vi "s3_bucket_demo.vi"() -> ()   [LabVIEW 2018]
uses:
  <vilib>/AWS Toolkit/Core/HTTP Request/Region.ctl
  <vilib>/AWS Toolkit/S3/ACL.ctl
  <vilib>/AWS Toolkit/S3/Bucket/Bucket.lvclass
  <vilib>/AWS Toolkit/Core/HTTP Request/AWS Credentials.ctl
  <vilib>/AWS Toolkit/Core/HTTP Request/HTTP Request.lvclass
  <vilib>/AWS Toolkit/S3/NI_AWS_S3.lvlib
panel:
  out "error constant":errorcluster
  out "Enum":T1(ring)
  in  "Stop":bool
  out "Owner display name":string
  out "Owner ID":string
  out "Buckets":refnum<class "Bucket.lvclass">[](array[class])
  in  "Access Control List":T2
  in  "Region":T3
  in  "Bucket Name":string
  in  "List":bool
  in  "Delete":bool
  in  "Create":bool
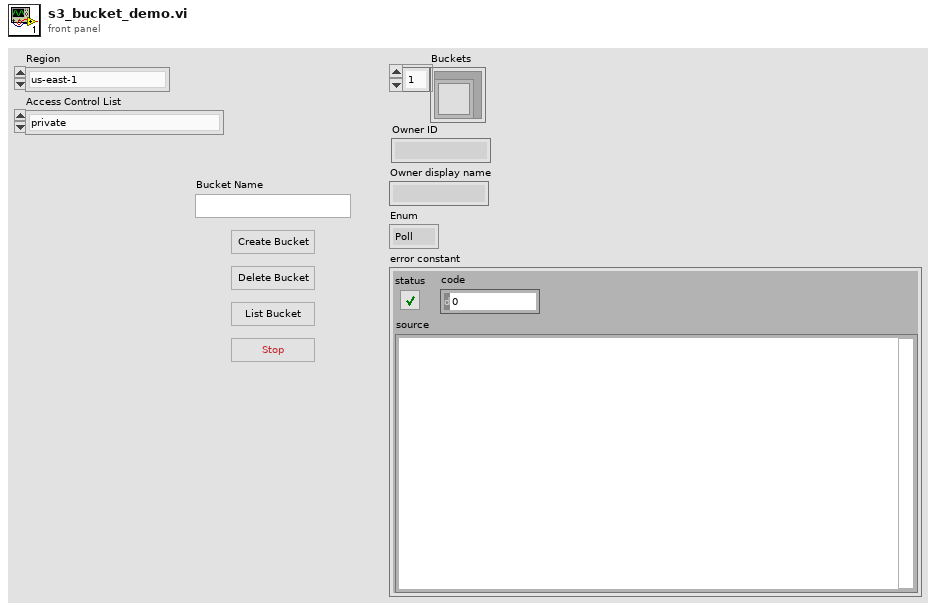
[diagram p1: front panel]
types:
  T1 = enum16{"Poll", "Create", "List", "Delete", "Shutdown"}
  T2 = typedef "NI_AWS_S3.lvlib/ACL.ctl" = enum16{"private", "public-read", "public-read-write", "aws-exec-read", "authenticated-read", "bucket-owner-read", "bucket-owner-full-control"}
  T3 = typedef "NI_AWS_Core.lvlib/HTTP Request.lvclass/Region.ctl" = enum16{"us-east-1", "us-east-2", "us-west-1", "us-west-2", "ap-northeast-1", "ap-northeast-2", "ap-southeast-1", "ap-southeast-2", "ca-central-1", "eu-central-1", "eu-west-1", "eu-west-2", "sa-east-1"}
  T4 = typedef "NI_AWS_Core.lvlib/HTTP Request.lvclass/AWS Credentials.ctl" = cluster{"Access Key":string, "Secret Key":string}
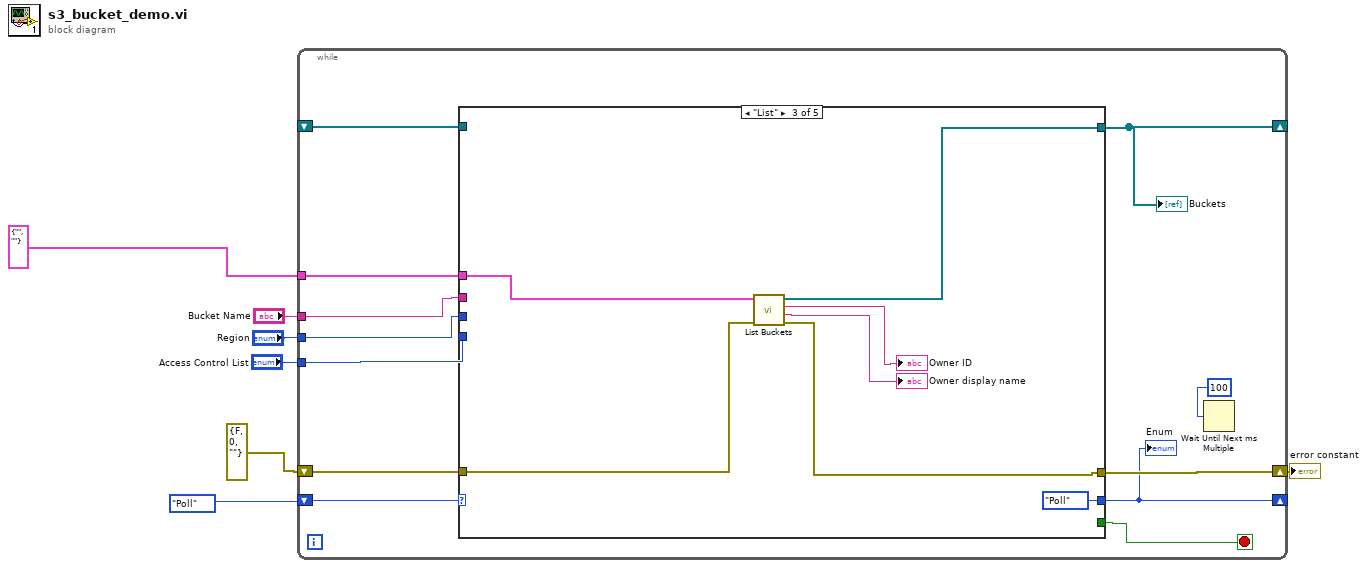
[diagram p0: block diagram]
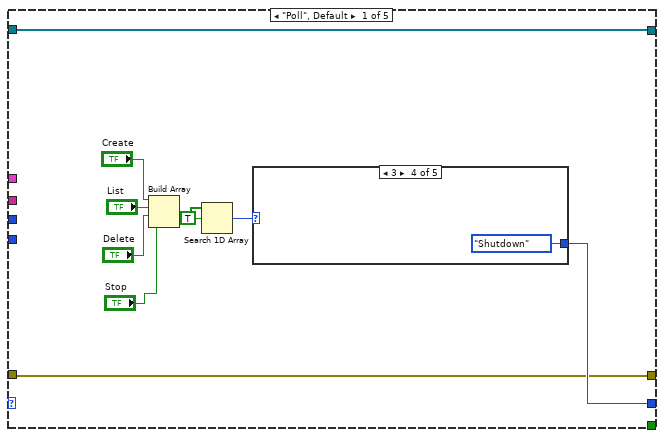
[diagram p2: hidden frame]
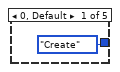
[diagram p3: hidden frame]
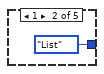
[diagram p4: hidden frame]
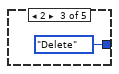
[diagram p5: hidden frame]
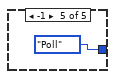
[diagram p6: hidden frame]
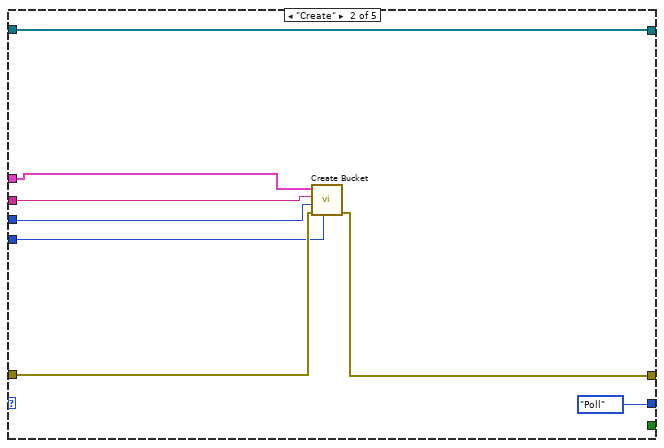
[diagram p7: hidden frame]
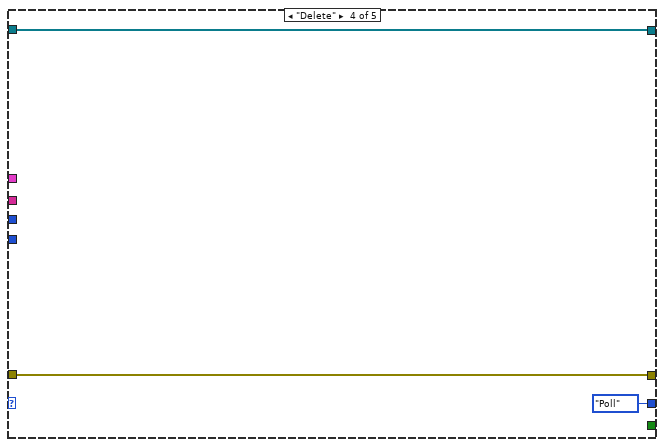
[diagram p8: hidden frame]
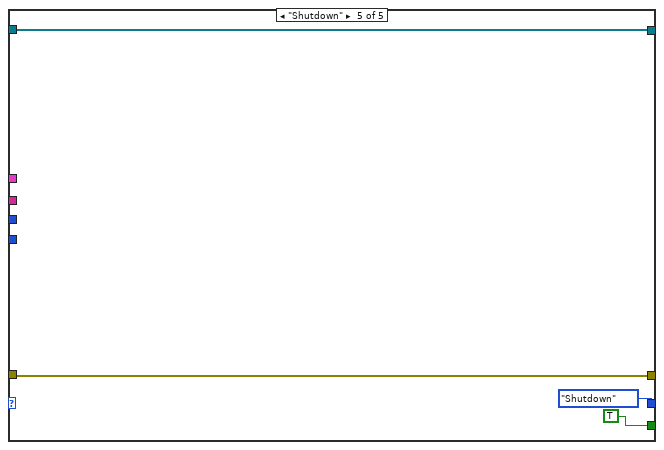
[diagram p9: hidden frame]
diagram:
  n1 = while {
    shift-right: [w8] -> _
    shift-left: T1."Poll" -> [w19]
    tunnel: T4 {"Access Key"="", "Secret Key"=""} ("AWS Credentials") -> [w17]
    tunnel: "Region" -> [w16]
    tunnel: "Bucket Name" -> [w15]
    shift-right: [w13] -> w1
    shift-left: errorcluster {"status"=FALSE, "code"=0, "source"=""} ("error constant") -> [w14]
    tunnel: "Access Control List" -> [w12]
    shift-right: [w11] -> _
    shift-left: _ -> [w10]
    stop <- w9 stop-if-true
    n2 = case shown="\"List\"" w19 {
      tunnel: [w23 T1."Poll" T1."Poll" T1."Poll" T1."Shutdown"] -> w8
      tunnel: w17 -> [_ w41 w49 _ _]
      tunnel: w16 -> [_ w40 _ _ _]
      tunnel: w15 -> [_ w39 _ _ _]
      tunnel: w14 -> [w22 w38 w48 w51 w54]
      tunnel: [w22 w37 w47 w51 w54] -> w13
      tunnel: w12 -> [_ w36 _ _ _]
      tunnel: [w20 w35 w46 w50 w53] -> w11
      tunnel: w10 -> [w20 w35 _ w50 w53]
      tunnel: [_ _ _ _ TRUE] -> w9
      frame "Poll", Default {
        n3 = Build Array("Create", "List", "Delete", "Stop") -> (w25:bool[])
        n4 = Search 1D Array(1D array=w25, element=TRUE) -> (index of element=w26:i32)  [unwired: 1 in]
        n5 = case shown="3" w26 {
          tunnel: [T1."Create" T1."List" T1."Delete" T1."Shutdown" T1."Poll"] -> w23
          frame 0, Default {
          }
          frame 1 {
          }
          frame 2 {
          }
          frame 3 {
          }
          frame -1 {
          }
        }
      }
      frame "Create" {
        n6 = call <vilib>:"Create Bucket.vi"("Access Control List"=w36, "error in (no error)"=w38, "Region"=w40, "Name"=w39, "AWS Credentials"=w41) -> ("error out"=w37:errorcluster)  [unwired: 5 in, 1 out]
      }
      frame "List" {
        n7 = call <vilib>:"List Buckets.vi"("error in (no error)"=w48, "AWS Credentials"=w49) -> ("error out"=w47:errorcluster, "Owner display name"=→"Owner display name":string, "Owner ID"=→"Owner ID":string, "Buckets"=w46:refnum<class "Bucket.lvclass">[])  [unwired: 6 in]
      }
      frame "Delete" {
      }
      frame "Shutdown" {
      }
    }
    "Buckets" <- w11
    "Enum" <- w8
    n8 = Wait Until Next ms Multiple(millisecond multiple=u32 100) -> ()  [unwired: 1 out]
  }
  "error constant" <- w1
